vi "Dashboard Main.vi"() -> ()   [LabVIEW 2014]
uses:
  <vilib>/event_ctls.llb/eventvkey.ctl
  <vilib>/Rock Robotics/WPI/Dashboard/WPI_DashboardLogging Global.vi
  <vilib>/Utility/config.llb/Write Key (String).vi
  <vilib>/Utility/config.llb/Write Key (I32).vi
  <vilib>/Utility/config.llb/NI_LVConfig.lvlib
panel:
  in  "Toggle":bool
  in  "Enable":bool
  in  "Axis Cam IP":string
  out "Camera IP 3":string
  out "Camera IP 2":string
  out "Small":T1(plugin-control)
  in  "TCP":refnum<k5>
  in  "Rec Mode":enum32{"Stop", "Record", "Playback"}(radio)
  in  "Vision":u16(ring) items=["Camera Off", "USB Camera SW", "USB Camera HW", "IP Camera"]
  out "Camera IP":string
  out "Image Message":string="Timeout in Camera Communications"
  in  "Dashboard Tab":T2(tab)
  in  "Backwards Driving":bool
  out "fps 2":dbl format="%#.1g"
  out "Mbps 4":dbl format="%#.1g"
  out "Mbps 3":bool
  in  "Camera Settings":T3={"Frame Rate"=30, "Compression"=30, "Size"=1} {"Frame Rate" scale=1.0..30.0; "Size" items=["640x480", "320x240", "160x120"]}
  out "MotorChart R":cluster{"Numeric":dbl, "Numeric":dbl}(graph)
  out "MotorChart L":T4(graph)
  out "MotorSliders R":cluster{"MotorSlide1":dbl, "MotorSlide2":dbl} {"MotorSlide2" scale=-1.0..1.0 scale format="%#_2e"; "MotorSlide1" scale=-1.0..1.0 scale format="%#_2e"}
  out "MotorSliders L":T5 {"MotorSlide4 2" scale=0.0..14.0 scale format="%#_2e"; "MotorSlide2" scale=-1.0..1.0 scale format="%#_2e"; "MotorSlide1" scale=-1.0..1.0 scale format="%#_2e"}
  out "Gyro":dbl(knob) scale=0.0..360.0
  out "JS1 Z":dbl(slide) scale=-1.0..1.0 scale format="%#_2e"
  out "JS1 Graph":cluster{"X":dbl, "Y":dbl}[](graph)
  out "JS1 Buttons":T6
  out "JS2 Z":dbl(slide) scale=-1.0..1.0 scale format="%#_2e"
  out "JS2 Graph":cluster{"X":dbl, "Y":dbl}[](graph)
  out "JS2 Buttons":T6
  out "Mode":T7(ring)=enum."Auto Disabled"
  in  "DB Camera Config":bool
  out "fps":dbl format="%#.1g"
  out "Mbps":dbl format="%#.1g"
  out "Mbps 2":bool
  in  "DB/String 9":string
  in  "DB/String 8":string
  in  "DB/String 7":string
  in  "DB/String 6":string
  in  "DB/String 5":string
  in  "DB/String 4":string
  in  "DB/String 3":string
  in  "DB/String 2":string
  in  "DB/String 1":string
  in  "DB/String 0":string
  in  "DB/Slider 0":dbl(slide) scale=0.0..5.0
  in  "DB/Slider 1":dbl(slide) scale=0.0..5.0
  in  "DB/Slider 2":dbl(slide) scale=0.0..5.0
  in  "DB/Slider 3":dbl(slide) scale=0.0..5.0
  out "DB/LED 3":bool
  out "DB/LED 2":bool
  out "DB/LED 1":bool
  out "DB/LED 0":bool
  in  "DB/Button 3":bool
  in  "DB/Button 2":bool
  in  "DB/Button 1":bool
  in  "DB/Button 0":bool caption="New Name"
  in  "Test Slider":dbl(slide) scale=0.0..100.0 scale format="%#_3g"
  in  "On/Off":bool caption="Solenoid"
  in  "Test Name":u16(ring) items=["Select the test to run...", "Example Test", "-------------------------------", "List of tests is built in robot code.", "Replace with your own automated tests."]
  in  "Test Tree":string(tree)
  in  "Motor":cluster{"Value":dbl, "Enable":bool} {"Value" scale=-1.0..1.0 scale format="%#_3g"}
  out "Progress":T8 {"Test Progress" scale=0.0..100.0}
  in  "Rev/Fwd":cluster{"Forward":bool, "Reverse":bool}
  in  "Test Ring":u16(ring) items=["Monochrome", "Color"]
  in  "Listbox":i32(listbox)
  out "Tree":string(tree)
  out "Big":T1(plugin-control)
  out "Boolean":bool
  # "Left"
  # "Front"
  # "Right"
  # "Battery"
  # "This tab is a great place for autonomous settings and robot-specific values.\nPlace controls and indicators inside this tab and match name to\nDashboard Variables on robot. You can also delete this comment."
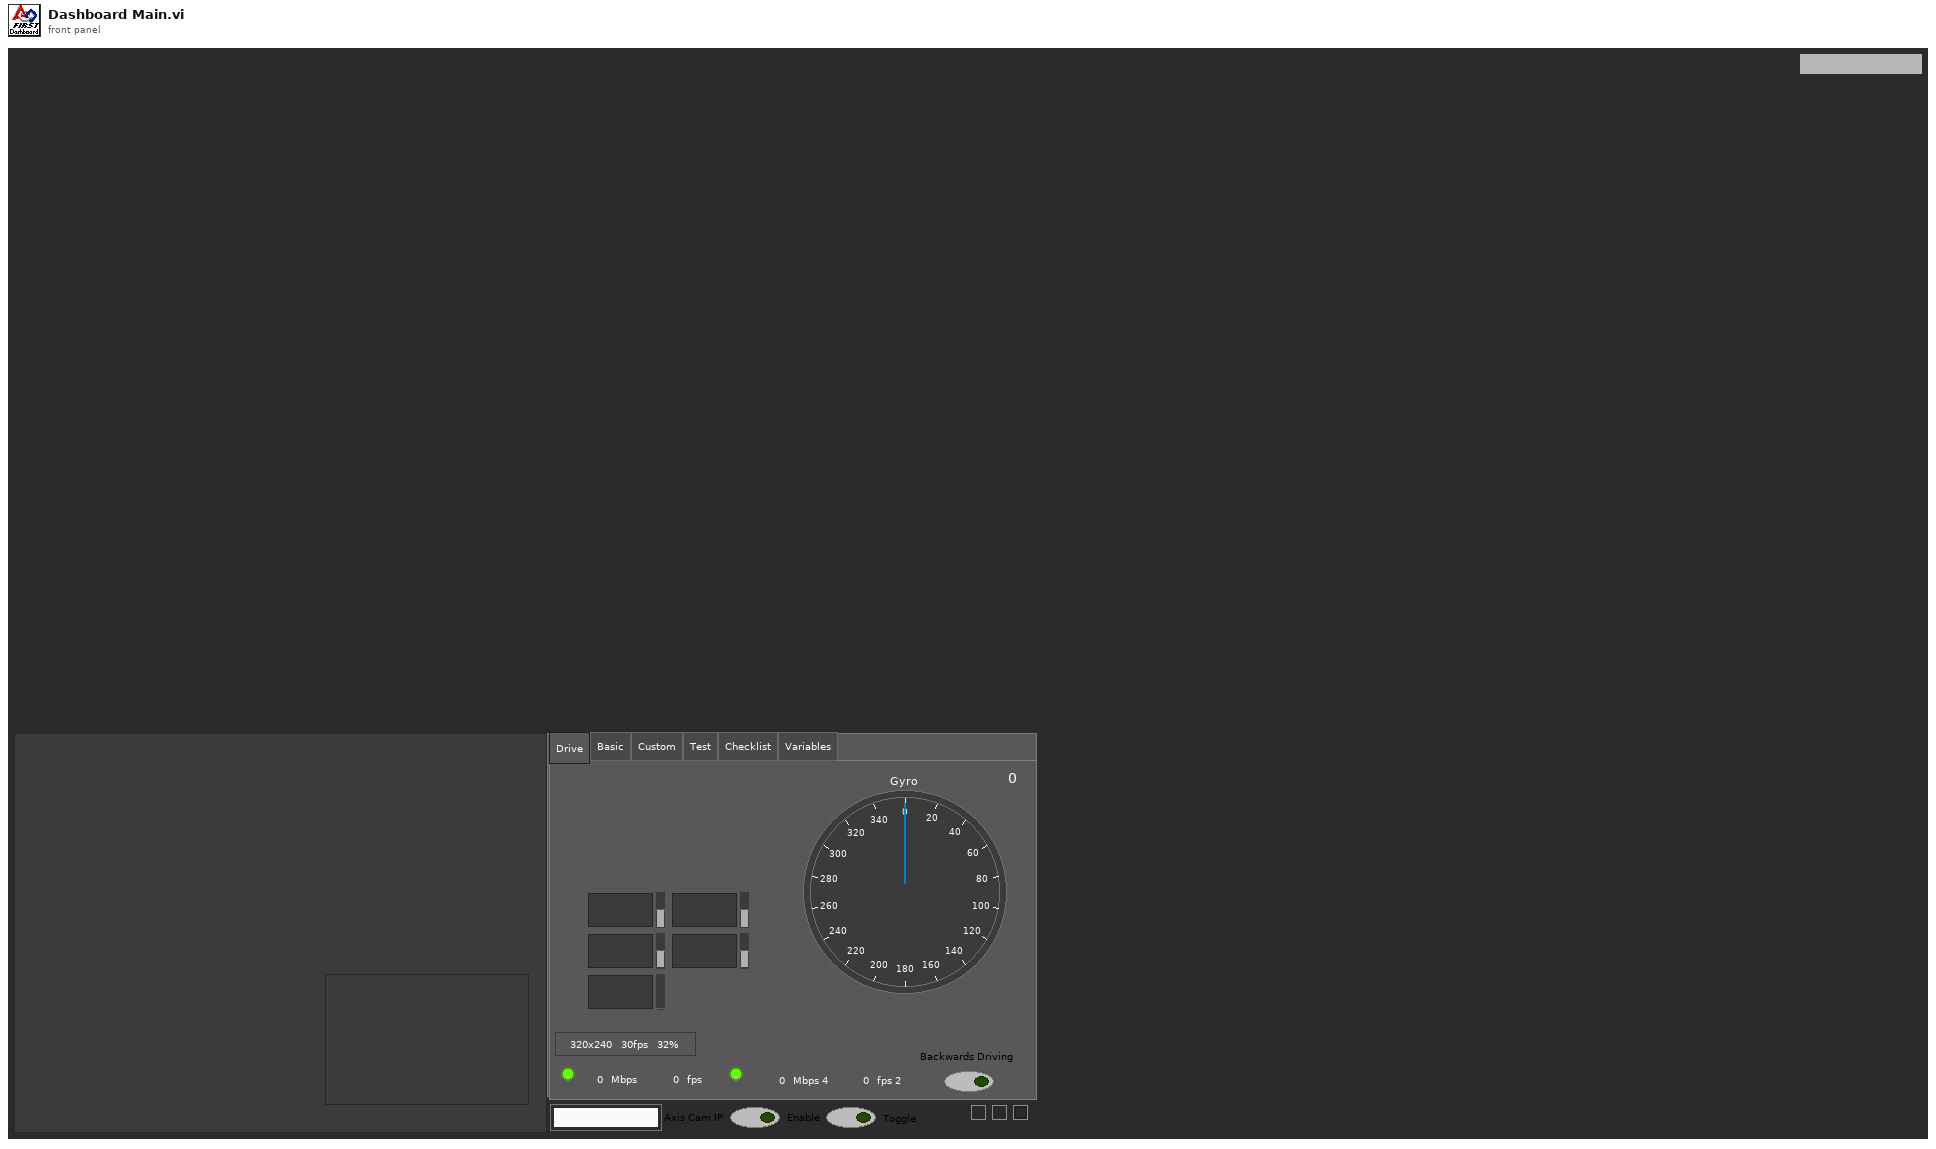
[diagram p1: front panel]
types:
  T1 = typedef "IMAQ Image.ctl" = refnum<image>
  T2 = enum32{"Drive", "Basic", "Custom", "Test", "Checklist", "Variables"}
  T3 = cluster{"Frame Rate":i32, "Compression":i32, "Size":u16}
  T4 = cluster{"Numeric":dbl, "Numeric":dbl, "Battery V":dbl}
  T5 = cluster{"MotorSlide1":dbl, "MotorSlide2":dbl, "MotorSlide4 2":dbl}
  T6 = cluster{bool, bool, bool, bool, bool, bool, bool, bool, bool, bool, bool, bool}
  T7 = enum8{"Tele-Op Disabled", "Tele-Op Enabled", "Auto Disabled", "Auto Enabled", "Test Disabled", "Test Enabled", "Disconnected", "No Code", "E-Stop"}
  T8 = cluster{"Test Progress":u8, "Test Progress Text":string}
  T9 = typedef "Image Type" = u32
  T10 = cluster{"Big":refnum<vi>, "Dashboard Tab":refnum<vi>, "Boolean":refnum<vi>, "Vision":refnum<vi>, "Rec Mode":refnum<vi>, "Test Slider":refnum<vi>, "On/Off ":refnum<vi>, "Test Ring":refnum<vi>, "Rev/Fwd":refnum<vi>, "Test Name":refnum<vi>, "Motor":refnum<vi>, "Progress":refnum<vi>, "CheckList":refnum<vi>, "Tree":refnum<vi>, "Test Tree":refnum<vi>}
  T11 = cluster{"Error Strings":string, "Disable Counts":cluster{u16, u16}, "Rail Faults":cluster{u16, u16, u16}, "Robot IP":string, "DB Mode":u8, "Event Info":cluster{"Name":string, "Type":u8, "Number":u16, "Replay":u8}, "Camera Addr":string}
  T12 = cluster{"Storage":cluster{"Disk Free":u64, "RAM Block":u32, "RAM free":u32}, "CPU Utilization":cluster{"CPU % ISR":sgl, "CPU % Time Crit":sgl, "CPU % Timed Str":sgl, "CPU % High":sgl, "CPU % Above":sgl, "CPU % Normal":sgl, "CPU % Low":sgl}, "CAN":cluster{"% Bus Utilization":sgl, "Bus Off Cnt":u32, "TX_FIFO Full Cnt":u32, "Receive Error Cnt":u8, "Transmit Error Cnt":u8}, "HID":cluster{"HID Outputs":u32, "Rumble Low":u16, "Rumble High":u16}[]}
  T13 = cluster{"Status bits":cluster{"Test Mode":bool, "Autonomous":bool, "Enabled":bool, "Code Start":bool, "Brownout":bool, "Reserved 2":bool, "Reserved 3":bool, "E-Stop":bool}, "Code Trace":cluster{"Disabled":bool, "TeleOp":bool, "Auto":bool, "Test":bool}, "Controller Type":enum16{"unknown", "cRIO", "roboRio"}, "Code?":enum16{"unknown", "noCode", "code"}, "Battery V":dbl}
  T14 = cluster{"Control Bits":cluster{"TestMode":bool, "Autonomous":bool, "Enabled":bool, "FMS Present":bool, bool, bool, bool, "E-Stop":bool}, "Team Station ":u8, "Countdown":sgl, "Joystick Values":cluster{"Axes":dbl[], "Buttons":bool[], "POVs":i16[]}[]}
  T15 = cluster{"Axes":dbl[], "Buttons":bool[], "POVs":i16[]}[]
  T16 = cluster{"Axes":dbl[], "Buttons":bool[], "POVs":i16[]}
  T17 = cluster{"Buttons[0]":bool, "Buttons[1]":bool, "Buttons[2]":bool, "Buttons[3]":bool, "Buttons[4]":bool, "Buttons[5]":bool, "Buttons[6]":bool, "Buttons[7]":bool, "Buttons[8]":bool, "Buttons[9]":bool, "Buttons[10]":bool, "Buttons[11]":bool}
  T18 = typedef "NI_LVConfig.lvlib/Config Data RefNum.ctl" = refnum<k1>
  T19 = cluster{"Operation":enum16{"Update", "Clear"}, "Color Box":u32}[]
  T20 = typedef "eventvkey.ctl" = enum16{"ASCII", "Enter", "Return", "Shift", "Ctrl", "Alt", "Cmd", "Opt", "Caps", "NumLock", "Clear", "Break", "Up", "Down", "Left", "Right", "Insert", "Delete", "Home", "End", "PageUp", "PageDown", "Escape", "Help", "Pause", "ScrollLock", "F1", "F2", "F3", "F4", "F5", "F6", "F7", "F8", "F9", "F10", "F11", "F12", "F13", "F14", "F15", "F16", "F17", "F18", "F19", "F20", "F21", "F22", "F23", "F24", "Play", "VolumeUp", "VolumeDown", "Mute", "Two Byte Char"}
  T21 = cluster{"Image Size":bool, "Image Type":bool, "Pixel Value":bool, "ROI Information":bool, "Zoom Factor":bool}
  T22 = enum8{"Enabled", "Disabled", "Disabled and Grayed Out"}
  T23 = cluster{"Operation":enum16{"Update", "Clear"}, "Color Box":u32}
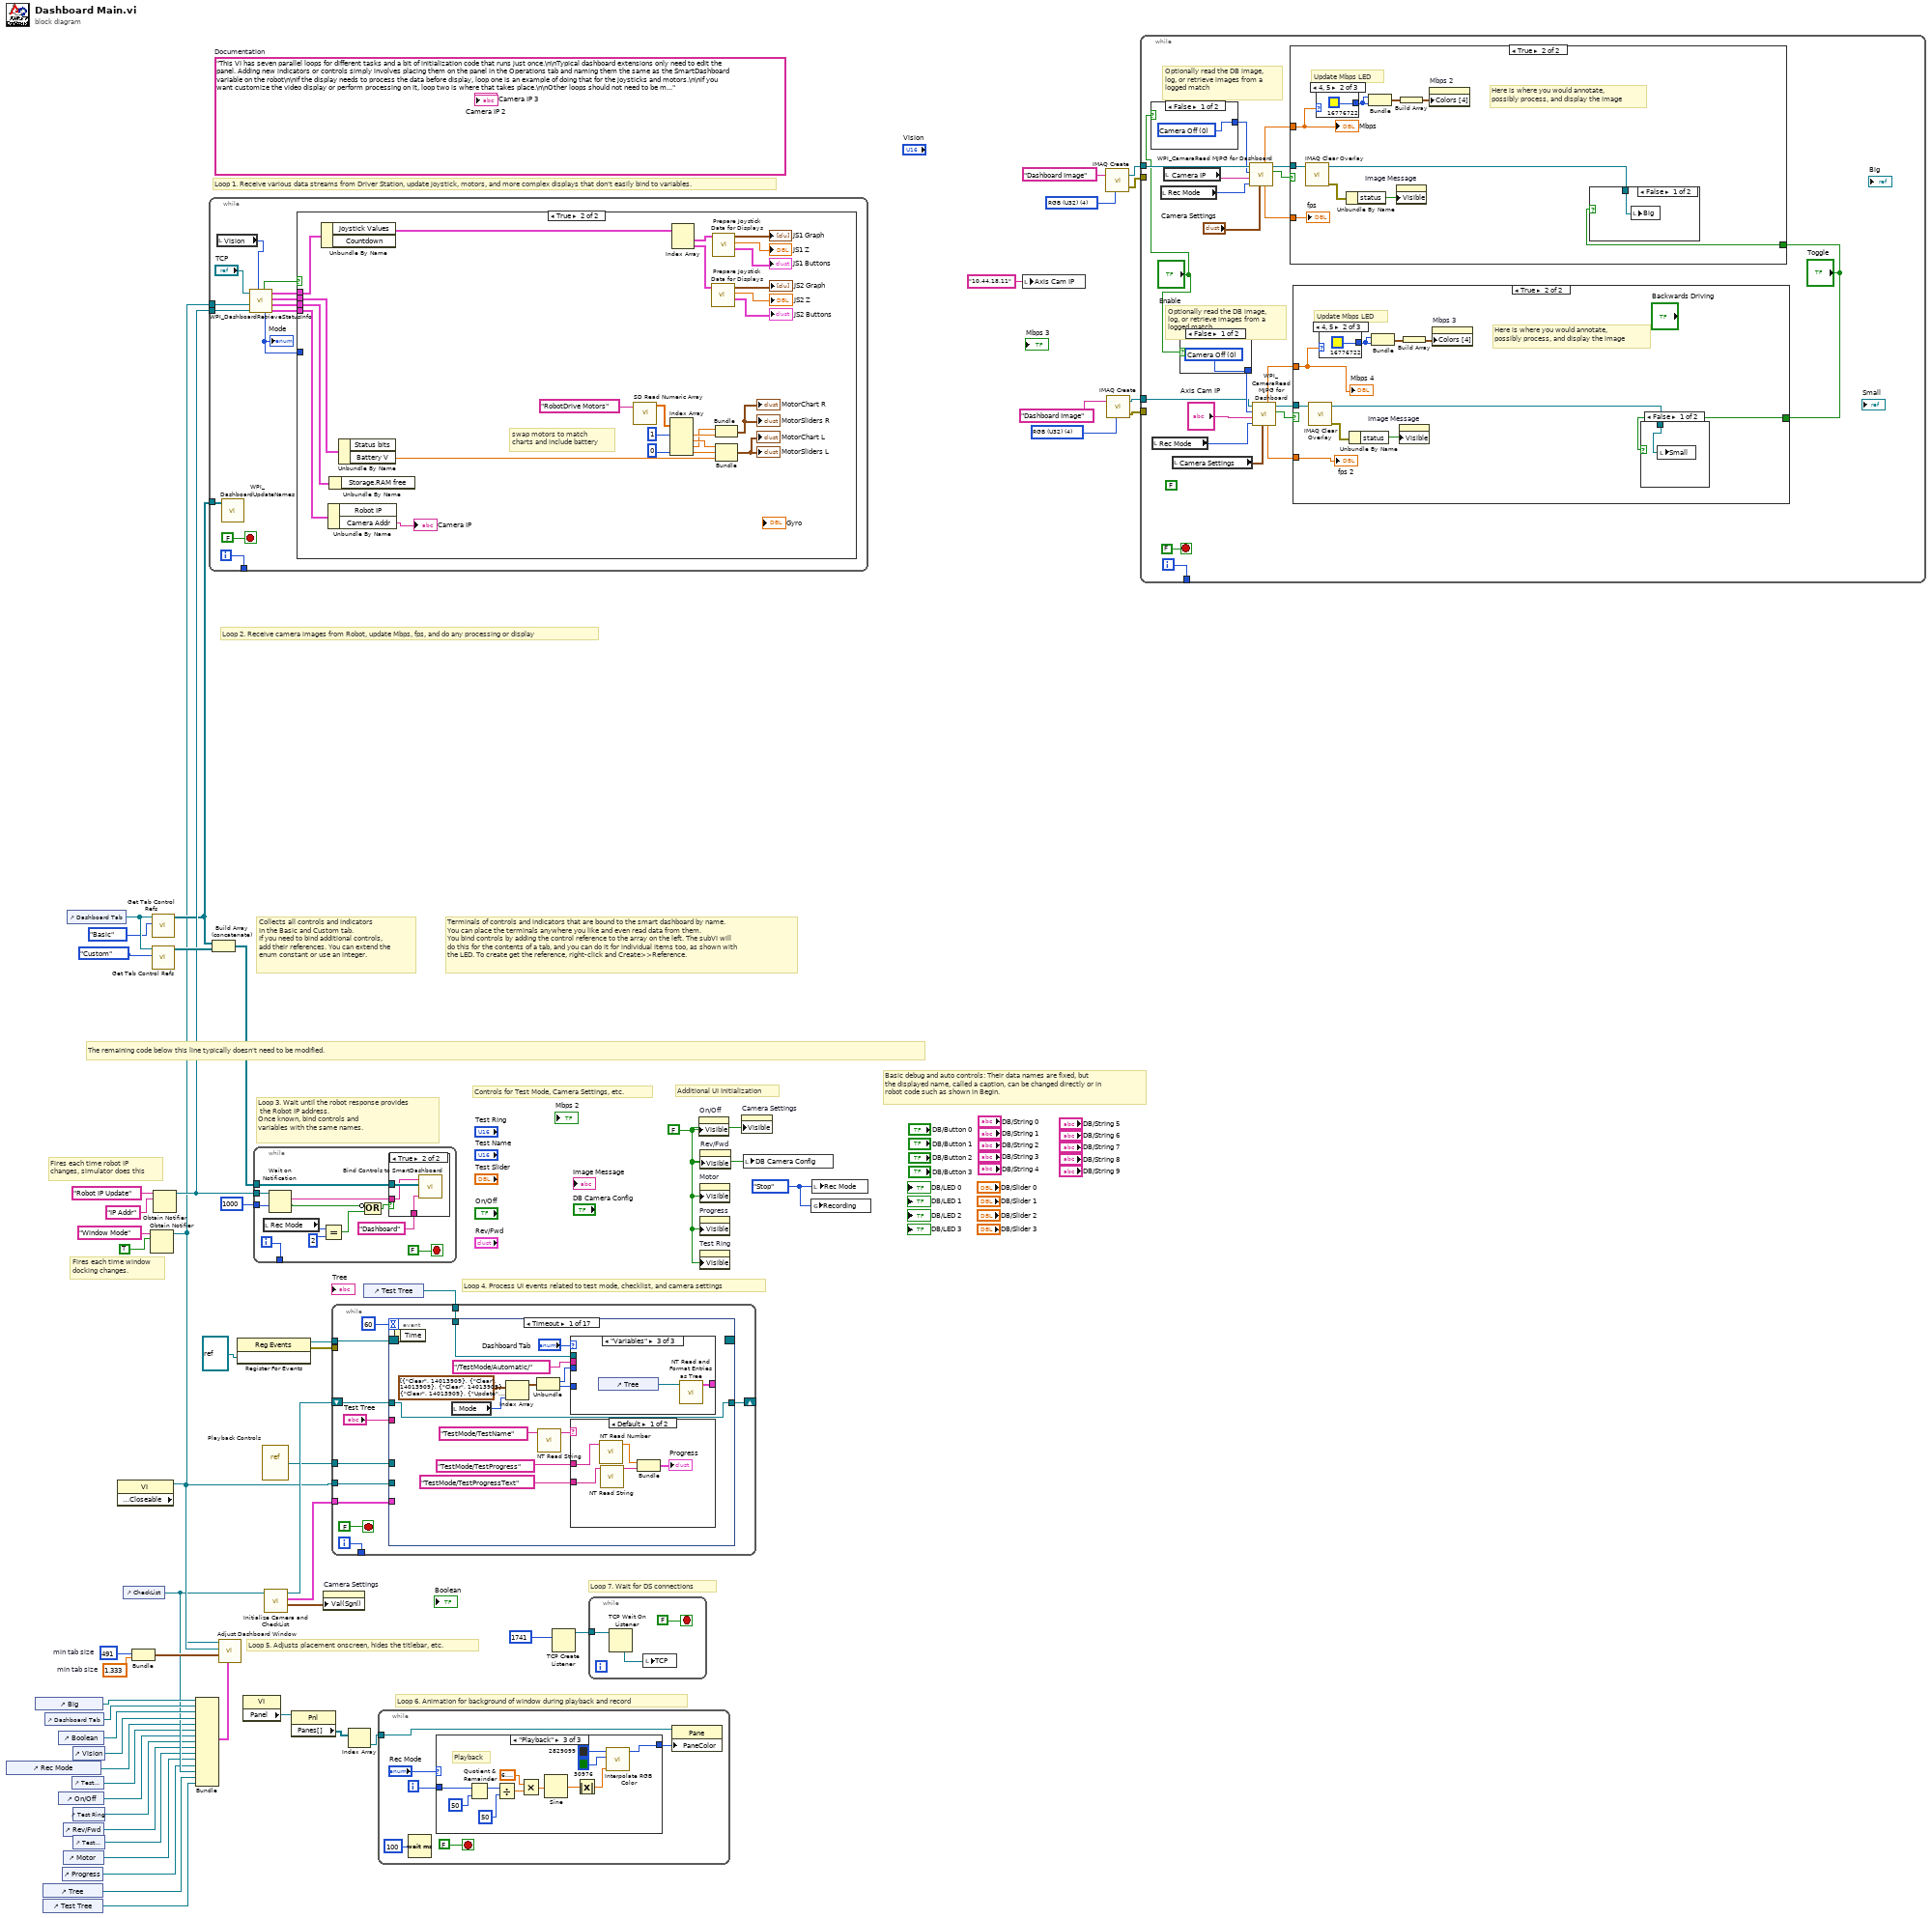
[diagram p0: block diagram]
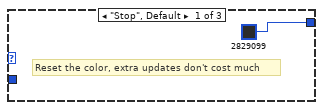
[diagram p3: hidden frame]
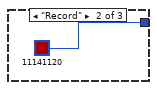
[diagram p4: hidden frame]
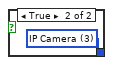
[diagram p6: hidden frame]
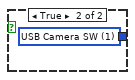
[diagram p7: hidden frame]
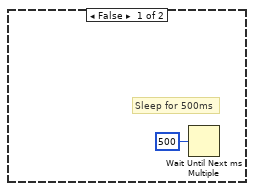
[diagram p8: hidden frame]
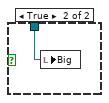
[diagram p9: hidden frame]
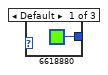
[diagram p10: hidden frame]
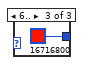
[diagram p11: hidden frame]
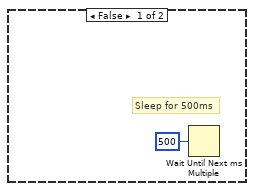
[diagram p12: hidden frame]
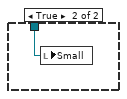
[diagram p13: hidden frame]
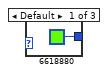
[diagram p14: hidden frame]
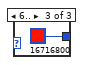
[diagram p15: hidden frame]
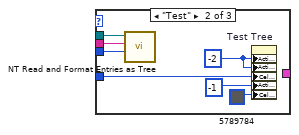
[diagram p17: hidden frame]
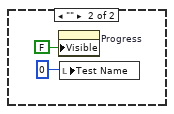
[diagram p18: hidden frame]
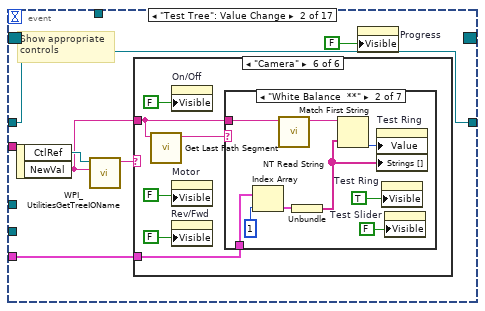
[diagram p19: hidden frame]
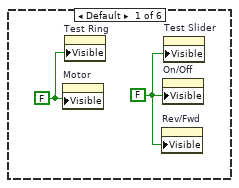
[diagram p20: hidden frame]
diagram:
  w4 = T9 4 items=["Grayscale (U8)", "Grayscale (I16)", "Grayscale (SGL)", "Complex (CSG)", "RGB (U32)", "HSL (U32)", "RGB (U64)"] ("Image Type")
  w29 = 491  # min tab size
  w28 = 1.333  # min tab size
  w37 = enum32{"Stop", "Record", "Playback"}."Stop" ("Rec Mode")
  w11 = FALSE ("Visible")
  (unwired) "This VI has seven parallel loops for different tasks and a bit of initialization code that runs just once.\n\nTypical dashboard extensions only need to edit the panel. Adding new indicators or controls simply involves placing them on the panel in the Operations tab and naming them the same as the SmartDashboard variable on the robot\n\nIf the display needs to process the data before display, loop one is an example of doing that for the joysticks and motors.\n\nIf you want customize the video display or perform processing on it, loop two is where that takes place.\n\nOther loops should not need to be modified. They are pretty standard, and document the task they perform."  # Documentation
  w57 = T9 4 items=["Grayscale (U8)", "Grayscale (I16)", "Grayscale (SGL)", "Complex (CSG)", "RGB (U32)", "HSL (U32)", "RGB (U64)"] ("Image Type")
  # "Loop 7. Wait for DS connections"
  # "Basic debug and auto controls: Their data names are fixed, but\nthe displayed name, called a caption, can be changed directly or in\nrobot code such as shown in Begin."
  # "Controls for Test Mode, Camera Settings, etc."
  # "Additional UI Initialization"
  # "Loop 6. Animation for background of window during playback and record"
  # "Fires each time robot IP\nchanges, simulator does this"
  # "Fires each time window\ndocking changes."
  # "Collects all controls and indicators\nin the Basic and Custom tab.\nIf you need to bind additional controls,\nadd their references. You can extend the\nenum constant or use an integer."
  # "The remaining code below this line typically doesn't need to be modified."
  # "Loop 4. Process UI events related to test mode, checklist, and camera settings"
  # "Terminals of controls and indicators that are bound to the smart dashboard by name.\nYou can place the terminals anywhere you like and even read data from them.\nYou bind controls by adding the control reference to the array on the left. The subVI will\ndo this for the contents of a tab, and you can do it for individual items too, as shown with\nthe LED. To create get the reference, right-click and Create>>Reference."
  # "Loop 3. Wait until the robot response provides\n the Robot IP address.\nOnce known, bind controls and\nvariables with the same names."
  # "Loop 5. Adjusts placement onscreen, hides the titlebar, etc."
  # "Loop 1. Receive various data streams from Driver Station, update joystick, motors, and more complex displays that don't easily bind to variables."
  # "Loop 2. Receive camera images from Robot, update Mbps, fps, and do any processing or display"
  n1 = control-ref of="Rec Mode"() -> (w17:refnum<vi>)
  n2 = control-ref of="Big"() -> (w32:refnum<vi>)
  n3 = control-ref of="Tree"() -> (w21:refnum<vi>)
  n4 = control-ref of="Test Tree"() -> (w20:refnum<vi>)
  n5 = control-ref of="Dashboard Tab"() -> (w31:refnum<vi>)
  n6 = control-ref of="Boolean"() -> (w26:refnum<vi>)
  n7 = control-ref of="On/Off"() -> (w15:refnum<vi>)
  n8 = control-ref of="Progress"() -> (w12:refnum<vi>)
  n9 = control-ref of="Rev/Fwd"() -> (w13:refnum<vi>)
  n10 = control-ref of="Motor"() -> (w18:refnum<vi>)
  n11 = control-ref of="Dashboard Tab"() -> (w35:refnum<vi>)
  n12 = control-ref of="Test Slider"() -> (w16:refnum<vi>)
  n13 = control-ref of="Vision"() -> (w30:refnum<vi>)
  n14 = control-ref of="Test Ring"() -> (w14:refnum<vi>)
  n15 = control-ref of="Test Name"() -> (w19:refnum<vi>)
  n16 = property class="VI" props=["Front Panel.Closeable"]() -> (reference out=w36:refnum<vi>)  [unwired: 2 in, 2 out]
  n17 = control-ref of="CheckList"() -> (w22:refnum<vi>)
  n18 = Bundle("min tab size"=w29, "min tab size"=w28) -> (w27:cluster{"min tab size":i32, "min tab size":dbl})  [unwired: 1 in]
  n19 = Obtain Notifier(name (unnamed)="Window Mode", notification data type=TRUE) -> (notifier out=w8:refnum<notifier>)  [unwired: 2 in, 2 out]
  n20 = call <vilib>:"Get Tab Control Refs.vi"("Page Index"=T2."Basic" ("Dashboard Tab"), "TabControl in"=w35) -> ("ControlsOnPage"=w9:refnum<vi>[])  [unwired: 9 in]
  n21 = call <vilib>:"Get Tab Control Refs.vi"("Page Index"=T2."Custom" ("Dashboard Tab"), "TabControl in"=w35) -> ("ControlsOnPage"=w34:refnum<vi>[])  [unwired: 9 in]
  n22 = Obtain Notifier(name (unnamed)="Robot IP Update", notification data type="IP Addr" ("name (unnamed)")) -> (notifier out=w10:refnum<notifier>)  [unwired: 2 in, 2 out]
  n23 = Bundle("Big"=w32, "Dashboard Tab"=w31, "Boolean"=w26, "Vision"=w30, "Rec Mode"=w17, "Test Slider"=w16, "On/Off"=w15, "Test Ring"=w14, "Rev/Fwd"=w13, "Test Name"=w19, "Motor"=w18, "Progress"=w12, "CheckList"=w22, "Tree"=w21, "Test Tree"=w20) -> (w23:T10)  [unwired: 1 in]
  n24 = while {
    tunnel: [w69] -> _
    tunnel: w10 -> [w63]
    tunnel: w9 -> [w62]
    tunnel: w8 -> [w58]
    i -> [w69]
    stop <- FALSE stop-if-true
    n25 = local read "Vision"() -> (w60:u16)
    n26 = call <vilib>:"WPI_DashboardUpdateNames.vi"("Controls on Tab"=w62) -> ()  [unwired: 11 in]
    n27 = call <vilib>:"WPI_DashboardRetrieveStatusInfo.vi"("Vision"=w60, "Binding Refnum"=w63, "Window Mode Notifier"=w58, "TCP Cnx"="TCP") -> ("Power and Errors"=w64:T11, "Robot Metrics"=w67:T12, "Status Info"=w68:T13, "Control Info"=w65:T14, "Robot Mode"=w61:T7, "Process?"=w66:bool)  [unwired: 2 in]
    "Mode" <- w61
    n28 = case shown="True" w66 {
      tunnel: w68 -> [_ w95]
      tunnel: w67 -> [_ w94]
      tunnel: w65 -> [_ w93]
      tunnel: w64 -> [_ w92]
      tunnel: w61 -> [_ _]
      frame False {
      }
      frame True {
        # "swap motors to match\ncharts and include battery"
        n29 = Unbundle By Name(w93) -> ("Joystick Values"=w80:T15)  [unwired: 1 out]
        n30 = Unbundle By Name(w92) -> ("Camera Addr"=→"Camera IP":string)  [unwired: 1 out]
        n31 = Unbundle By Name(w94) -> ()  [unwired: 1 out]
        n32 = Unbundle By Name(w95) -> ("Battery V"=w81:dbl)  [unwired: 1 out]
        n33 = call <vilib>:"SD Read Numeric Array.vi"("Name"="RobotDrive Motors") -> ("Numeric Array"=w83:dbl[])  [unwired: 8 in, 2 out]
        n34 = Index Array(array=w83, index #1=1, index #4=0) -> (element #1=w87:dbl, element #2=w88:dbl, element #3=w86:dbl, element #4=w91:dbl)  [unwired: 2 in]
        n35 = Index Array(array=w80) -> (element #1=w79:T16, element #2=w74:T16)  [unwired: 2 in]
        n36 = call "Prepare Joystick Data for Displays.vi"("Joystick Values"=w74) -> ("Buttons"=→"JS2 Buttons":T17, "Z Axis"=→"JS2 Z":dbl, "Cartesian Data"=→"JS2 Graph":cluster{"X axis":dbl, "X axis":dbl}[])  [unwired: 8 in]
        n37 = call "Prepare Joystick Data for Displays.vi"("Joystick Values"=w79) -> ("Buttons"=→"JS1 Buttons":T17, "Z Axis"=→"JS1 Z":dbl, "Cartesian Data"=→"JS1 Graph":cluster{"X axis":dbl, "X axis":dbl}[])  [unwired: 8 in]
        n38 = Bundle("Numeric"=w86, "Numeric"=w87) -> (→"MotorChart R" →"MotorSliders R":cluster{"Numeric":dbl, "Numeric":dbl})  [unwired: 1 in]
        n39 = Bundle("Numeric"=w88, "Numeric"=w91, "Battery V"=w81) -> (→"MotorChart L" →"MotorSliders L":T4)  [unwired: 1 in]
      }
    }
  }
  n40 = Build Array (concatenate)(w9, w34) -> (w33:refnum<vi>[])
  n41 = call "Adjust Dashboard Window.vi"("Sizing Refnums"=w23, "Size Constraints"=w27, "VI"=w36, "Notifier in"=w8) -> ()  [unwired: 8 in]
  n42 = register-events(refnum<vi> refnum) -> (reference out=w41:refnum<event-registration>, error out=w40:errorcluster)  [unwired: 2 in]
  n43 = property class="VI"() -> ("Panel"=w44:refnum<vi>)  [unwired: 2 in, 2 out]
  n44 = while {
    tunnel: w33 -> [w107]
    tunnel: w10 -> [w105]
    tunnel: [w103] -> _
    tunnel: u32 1000 ("milliseconds to wait") -> [w102]
    i -> [w103]
    stop <- FALSE stop-if-true
    n45 = local read "Rec Mode"() -> (w98:enum32{"Stop", "Record", "Playback"})
    n46 = Wait on Notification(notifier=w105, timeout in ms (-1)=w102) -> (notification=w104:string, timed out?=w100:bool)  [unwired: 2 in, 2 out]
    n47 = Equal?(x=w98, y=u16 2 ("Rec Mode")) -> (x = y?=w99:bool)
    n48 = Compound Arithmetic op=OR(invert w100, w99) -> (w101:bool)
    n49 = case shown="True" w101 {
      tunnel: w107 -> [_ w110]
      tunnel: w104 -> [_ w109]
      tunnel: "Dashboard" -> [_ w108]
      frame False {
      }
      frame True {
        n50 = call <vilib>:"Bind Controls to SmartDashboard.vi"("Client Name"=w108, "Bound Control Refs"=w110, "Server IP Address"=w109) -> ()  [unwired: 9 in]
      }
    }
  }
  n51 = vi-ref "Playback Controls.vi"() -> (w42:refnum<vi>)
  n52 = call "Initialize Camera and CheckList.vi"("ListBox in"=w22) -> ("Cluster"=w48:cluster{"value":i32, "value":i32, "index":i32}, "Array"=w49:cluster{string[]}[], "File Refnum"=w47:T18)  [unwired: 8 in]
  n53 = property class="Pnl"(reference=w44) -> ("Panes[]"=w45:refnum<vi>[])  [unwired: 1 in, 2 out]
  n54 = property on="Camera Settings" class="Clust (strict)"("Val(Sgnl)"=w48) -> ()  [unwired: 2 in, 2 out]
  n55 = Index Array(array=w45) -> (element=w43:refnum<vi>)  [unwired: 1 in]
  n56 = control-ref of="Test Tree"() -> (w46:refnum<vi>)
  n57 = while {
    tunnel: w49 -> [w118]
    shift-right: [w117] -> _
    shift-left: w47 -> [w116]
    tunnel: [w115] -> _
    tunnel: w46 -> [w114]
    tunnel: w42 -> [w113]
    tunnel: w41 -> [w112]
    tunnel: w40 -> [_]
    tunnel: w36 -> [w111]
    i -> [w115]
    stop <- FALSE stop-if-true
    n58 = event shown="[0] Timeout" {
      selector: w112 -> [_ _ _ _ _ _ _ _ _ _ _ _ _ _ _ _ _]
      dyn-events: [_ _ _ _ _ _ _ _ _ _ _ _ _ w356 _ _ _] -> _
      timeout: u32 60 ("milliseconds to wait") -> [_ _ _ _ _ _ _ _ _ _ _ _ _ _ _ _ _]
      tunnel: w114 -> [w130 _ _ _ _ _ _ _ _ _ _ _ _ _ _ _ _]
      tunnel: "Test Tree" -> [_ _ _ _ _ _ _ _ w325 w333 w335 w339 w347 _ _ _ _]
      tunnel: w118 -> [_ w152 _ _ _ _ w289 w319 _ _ _ _ _ _ _ _ _]
      tunnel: [w126 w151 w250 w255 w263 w275 w288 w312 w324 w331 w334 w338 w346 w358 w372 w373 w383] -> w117
      tunnel: w116 -> [w126 w151 w250 w255 w263 w275 w287 w312 w324 w331 w334 w338 w346 w358 w372 w373 w383]
      tunnel: w113 -> [_ _ _ _ _ _ _ _ _ _ _ _ _ w359 _ w376 _]
      tunnel: w111 -> [_ _ _ _ _ _ _ _ _ _ _ _ _ w354 _ _ _]
      event Timeout {
        n59 = event-data() -> ()  [unwired: 1 in, 1 out]
        n60 = local read "Mode"() -> (w129:T7)
        n61 = Index Array(array=T19 [{"Operation"=enum."Clear", "Color Box"=14013909}, {"Operation"=enum."Clear", "Color Box"=14013909}, {"Operation"=enum."Clear", "Color Box"=14013909}, {"Operation"=enum."Clear", "Color Box"=14013909}, {"Operation"=enum."Update", "Color Box"=14013909}, {"Operation"=enum."Update", "Color Box"=16777215}, {"Operation"=enum."Clear", "Color Box"=14013909}, {"Operation"=enum."Clear", "Color Box"=14013909}, {"Operation"=enum."Clear", "Color Box"=14013909}], index=w129) -> (element=w124:T23)
        n62 = Unbundle(w124) -> ("Operation"=w123:enum16{"Update", "Clear"}, "Color Box"=w122:u32)
        n63 = call <vilib>:"NT Read String.vi"("Name"="TestMode/TestName") -> ("String"=w133:string)  [unwired: 9 in, 1 out]
        n64 = case shown="\"Variables\"" "Dashboard Tab" {
          tunnel: w130 -> [_ w141 _]
          tunnel: "/TestMode/Automatic/" ("Name Pattern") -> [_ w140 _]
          tunnel: w123 -> [_ w139 _]
          tunnel: [_ _ w143] -> _
          tunnel: w122 -> [_ w135 _]
          frame "Custom", Default {
          }
          frame "Test" {
            w138 = -2 ("Active Item:Row Number")
            n65 = call <vilib>:"NT Read and Format Entries as Tree.vi"("Operation"=w139, "Name Pattern"=w140, "Tree Refnum"=w141) -> ()  [unwired: 7 in, 2 out]
            n66 = property on="Test Tree" class="Tree (strict)"("Active Item Row Number"=w138, "ActiveColNum"=w138, "CellBG"=w135, "Active Item Row Number"=-1 ("Active Item:Row Number"), "CellBG"=u32 5789784 ("Color Box")) -> ()  [unwired: 2 in, 2 out]
          }
          frame "Variables" {
            n67 = control-ref of="Tree"() -> (w142:refnum<vi>)
            n68 = call <vilib>:"NT Read and Format Entries as Tree.vi"("Tree Refnum"=w142) -> ("Formatted Strings"=w143:cluster{"Name":string, "Value":string}[])  [unwired: 9 in, 1 out]
          }
        }
        n69 = case shown="Default" w133 {
          tunnel: "TestMode/TestProgress" ("Name") -> [w145 _]
          tunnel: "TestMode/TestProgressText" ("Name") -> [w144 _]
          frame Default {
            n70 = call <vilib>:"NT Read Number.vi"("Name"=w145) -> ("Numeric"=w146:dbl)  [unwired: 9 in, 1 out]
            n71 = call <vilib>:"NT Read String.vi"("Name"=w144) -> ("String"=w147:string)  [unwired: 9 in, 1 out]
            n72 = Bundle("Numeric"=w146, "String"=w147) -> (→"Progress":cluster{"Numeric":dbl, "String":string})  [unwired: 1 in]
          }
          frame "" {
            n73 = property on="Progress" class="Clust (strict)"("Visible"=FALSE) -> ()  [unwired: 2 in, 2 out]
            n74 = local write "Test Name"(u16 0) -> ()
          }
        }
      }
      event "Test Tree": Value Change {
        # "Show appropriate\ncontrols"
        n75 = event-data() -> ("CtlRef"=w155:refnum<vi>, "NewVal"=w153:string)  [unwired: 1 in]
        n76 = call <vilib>:"WPI_UtilitiesGetTreeIOName.vi"("NewVal"=w153, "TreeControl in"=w155) -> ("I/O Name"=w156:string)  [unwired: 9 in]
        n77 = case shown="\"Camera\"" w156 {
          selector: w156 -> [_ w163 _ w181 w190 _]
          tunnel: w153 -> [_ _ w178 w180 _ w197]
          tunnel: w152 -> [_ _ _ _ _ w196]
          frame Default {
            w158 = FALSE ("Visible")
            w157 = FALSE ("Visible")
            n78 = property on="Motor" class="Clust (strict)"("Visible"=w157) -> ()  [unwired: 2 in, 2 out]
            n79 = property on="Test Ring" class="Ring (strict)"("Visible"=w157) -> ()  [unwired: 2 in, 2 out]
            n80 = property on="Rev/Fwd" class="Clust (strict)"("Visible"=w158) -> ()  [unwired: 2 in, 2 out]
            n81 = property on="On/Off" class="Bool (strict)"("Visible"=w158) -> ()  [unwired: 2 in, 2 out]
            n82 = property on="Test Slider" class="Slide (strict)"("Visible"=w158) -> ()  [unwired: 2 in, 2 out]
          }
          frame "Motor", "PWM" {
            w164 = FALSE ("Visible")
            n83 = case shown="\"Motor\", Default" w163 {
              tunnel: [1.0 ("Value") -1.0 ("Value")] -> w162
              tunnel: [255.0 ("Value") 1.0 ("Value")] -> w161
              tunnel: [128.0 ("Value") 0.0 ("Value")] -> w160
              tunnel: [64.0 ("Value") 0.5 ("Value")] -> w159
              frame "PWM" {
              }
              frame "Motor", Default {
              }
            }
            n84 = property on="Motor" class="Clust (strict)"("Visible"=TRUE) -> ()  [unwired: 2 in, 2 out]
            n85 = property on="Value" class="Slide (strict)"("Value"=w160, "Scale.Minimum"=w162, "Scale.Maximum"=w161, "Scale.Increment"=w159) -> ()  [unwired: 2 in, 2 out]
            n86 = property on="On/Off" class="Bool (strict)"("Visible"=w164) -> ()  [unwired: 2 in, 2 out]
            n87 = property on="Test Slider" class="Slide (strict)"("Visible"=w164) -> ()  [unwired: 2 in, 2 out]
            n88 = property on="Test Ring" class="Ring (strict)"("Visible"=w164) -> ()  [unwired: 2 in, 2 out]
            n89 = property on="Rev/Fwd" class="Clust (strict)"("Visible"=w164) -> ()  [unwired: 2 in, 2 out]
          }
          frame "Servo" {
            w176 = FALSE ("Visible")
            n90 = call <vilib>:"NT Read Number.vi"("Name"=w178) -> ("Numeric"=w177:dbl)  [unwired: 9 in, 1 out]
            n91 = property on="Test Slider" class="Slide (strict)"("Visible"=TRUE, "Scale.Maximum"=170.0 ("Scale.Range:Maximum")) -> ()  [unwired: 2 in, 2 out]
            n92 = local write "Test Slider"(w177) -> ()
            n93 = property on="Motor" class="Clust (strict)"("Visible"=w176) -> ()  [unwired: 2 in, 2 out]
            n94 = property on="Rev/Fwd" class="Clust (strict)"("Visible"=w176) -> ()  [unwired: 2 in, 2 out]
            n95 = property on="On/Off" class="Bool (strict)"("Visible"=w176) -> ()  [unwired: 2 in, 2 out]
            n96 = property on="Test Ring" class="Ring (strict)"("Visible"=w176) -> ()  [unwired: 2 in, 2 out]
          }
          frame "Relay", "Solenoid" {
            w179 = FALSE ("Visible")
            n97 = property on="Motor" class="Clust (strict)"("Visible"=w179) -> ()  [unwired: 2 in, 2 out]
            n98 = property on="Test Slider" class="Slide (strict)"("Visible"=w179) -> ()  [unwired: 2 in, 2 out]
            n99 = Search and Replace String(input string=w180, search string="/Value  **", replace string="/Direction") -> (result string=w186:string)  [unwired: 5 in, 3 out]
            n100 = property on="Test Ring" class="Ring (strict)"("Visible"=w179) -> ()  [unwired: 2 in, 2 out]
            n101 = call <vilib>:"NT Read String.vi"("Name"=w186) -> ("String"=w184:string)  [unwired: 9 in, 1 out]
            n102 = Equal?(x="Both directions", y=w184) -> (x = y?=w182:bool)
            n103 = Not(x=w182) -> (.not. x?=w183:bool)
            n104 = property on="Rev/Fwd" class="Clust (strict)"("Visible"=w182) -> ()  [unwired: 2 in, 2 out]
            n105 = property on="On/Off" class="Bool (strict)"("Visible"=w183, "Caption.Text"=w181) -> ()  [unwired: 2 in, 2 out]
          }
          frame "Compressor", "Digital Out" {
            w189 = FALSE ("Visible")
            # "Get direction and finish"
            n106 = property on="Motor" class="Clust (strict)"("Visible"=w189) -> ()  [unwired: 2 in, 2 out]
            n107 = property on="Test Slider" class="Slide (strict)"("Visible"=w189) -> ()  [unwired: 2 in, 2 out]
            n108 = property on="Test Ring" class="Ring (strict)"("Visible"=w189) -> ()  [unwired: 2 in, 2 out]
            n109 = property on="On/Off" class="Bool (strict)"("Visible"=TRUE, "Caption.Text"=w190) -> ()  [unwired: 2 in, 2 out]
            n110 = property on="Rev/Fwd" class="Clust (strict)"("Visible"=FALSE) -> ()  [unwired: 2 in, 2 out]
          }
          frame "Camera" {
            n111 = call <vilib>:"Get Last Path Segment.vi"("String in"=w197) -> ("String out"=w198:string)  [unwired: 10 in]
            n112 = property on="On/Off" class="Bool (strict)"("Visible"=FALSE) -> ()  [unwired: 2 in, 2 out]
            n113 = property on="Motor" class="Clust (strict)"("Visible"=FALSE) -> ()  [unwired: 2 in, 2 out]
            n114 = property on="Rev/Fwd" class="Clust (strict)"("Visible"=FALSE) -> ()  [unwired: 2 in, 2 out]
            n115 = case shown="\"White Balance  **\"" w198 {
              tunnel: w197 -> [w204 w213 w222 w231 w240 _ w246]
              tunnel: w196 -> [w202 w210 w219 w228 w237 _ _]
              frame "Size  **" {
                n116 = Index Array(array=w202) -> (element=w201:cluster{string[]})  [unwired: 1 in]
                n117 = call <vilib>:"NT Read String.vi"("Name"=w204) -> ("String"=w203:string)  [unwired: 9 in, 1 out]
                n118 = Unbundle(w201) -> (w199:string[])
                n119 = Match First String(2:w199, 3:w203) -> (0:w200:i32)  [unwired: 1 out]
                n120 = property on="Test Ring" class="Ring (strict)"("Value"=w200, "Strings []"=w199) -> ()  [unwired: 2 in, 2 out]
                n121 = property on="Test Ring" class="Ring (strict)"("Visible"=TRUE) -> ()  [unwired: 2 in, 2 out]
                n122 = property on="Test Slider" class="Slide (strict)"("Visible"=FALSE) -> ()  [unwired: 2 in, 2 out]
              }
              frame "White Balance  **" {
                n123 = Index Array(array=w210, index=1) -> (element=w211:cluster{string[]})
                n124 = call <vilib>:"NT Read String.vi"("Name"=w213) -> ("String"=w212:string)  [unwired: 9 in, 1 out]
                n125 = Unbundle(w211) -> (w208:string[])
                n126 = Match First String(2:w208, 3:w212) -> (0:w207:i32)  [unwired: 1 out]
                n127 = property on="Test Ring" class="Ring (strict)"("Value"=w207, "Strings []"=w208) -> ()  [unwired: 2 in, 2 out]
                n128 = property on="Test Ring" class="Ring (strict)"("Visible"=TRUE) -> ()  [unwired: 2 in, 2 out]
                n129 = property on="Test Slider" class="Slide (strict)"("Visible"=FALSE) -> ()  [unwired: 2 in, 2 out]
              }
              frame "Exposure  **" {
                n130 = Index Array(array=w219, index=2) -> (element=w220:cluster{string[]})
                n131 = call <vilib>:"NT Read String.vi"("Name"=w222) -> ("String"=w221:string)  [unwired: 9 in, 1 out]
                n132 = Unbundle(w220) -> (w216:string[])
                n133 = Match First String(2:w216, 3:w221) -> (0:w217:i32)  [unwired: 1 out]
                n134 = property on="Test Ring" class="Ring (strict)"("Value"=w217, "Strings []"=w216) -> ()  [unwired: 2 in, 2 out]
                n135 = property on="Test Ring" class="Ring (strict)"("Visible"=TRUE) -> ()  [unwired: 2 in, 2 out]
                n136 = property on="Test Slider" class="Slide (strict)"("Visible"=FALSE) -> ()  [unwired: 2 in, 2 out]
              }
              frame "Exposure Priority  **" {
                n137 = Index Array(array=w228, index=3) -> (element=w229:cluster{string[]})
                n138 = call <vilib>:"NT Read String.vi"("Name"=w231) -> ("String"=w230:string)  [unwired: 9 in, 1 out]
                n139 = Unbundle(w229) -> (w225:string[])
                n140 = Match First String(2:w225, 3:w230) -> (0:w226:i32)  [unwired: 1 out]
                n141 = property on="Test Ring" class="Ring (strict)"("Value"=w226, "Strings []"=w225) -> ()  [unwired: 2 in, 2 out]
                n142 = property on="Test Ring" class="Ring (strict)"("Visible"=TRUE) -> ()  [unwired: 2 in, 2 out]
                n143 = property on="Test Slider" class="Slide (strict)"("Visible"=FALSE) -> ()  [unwired: 2 in, 2 out]
              }
              frame "Color Enable  **" {
                n144 = Index Array(array=w237, index=4) -> (element=w238:cluster{string[]})
                n145 = call <vilib>:"NT Read String.vi"("Name"=w240) -> ("String"=w239:string)  [unwired: 9 in, 1 out]
                n146 = Unbundle(w238) -> (w234:string[])
                n147 = Match First String(2:w234, 3:w239) -> (0:w235:i32)  [unwired: 1 out]
                n148 = property on="Test Ring" class="Ring (strict)"("Value"=w235, "Strings []"=w234) -> ()  [unwired: 2 in, 2 out]
                n149 = property on="Test Ring" class="Ring (strict)"("Visible"=TRUE) -> ()  [unwired: 2 in, 2 out]
                n150 = property on="Test Slider" class="Slide (strict)"("Visible"=FALSE) -> ()  [unwired: 2 in, 2 out]
              }
              frame Default {
                n151 = property on="Test Ring" class="Ring (strict)"("Visible"=FALSE) -> ()  [unwired: 2 in, 2 out]
                n152 = property on="Test Slider" class="Slide (strict)"("Visible"=FALSE) -> ()  [unwired: 2 in, 2 out]
              }
              frame "Brightness  **", "Color Level  **", "Compression  **", "FPS  **", "Sharpness  **" {
                n153 = call <vilib>:"NT Read Number.vi"("Name"=w246) -> ("Numeric"=w245:dbl)  [unwired: 9 in, 1 out]
                n154 = local write "Test Slider"(w245) -> ()
                n155 = property on="Test Slider" class="Slide (strict)"("Visible"=TRUE, "Scale.Maximum"=100.0 ("Scale.Range:Maximum")) -> ()  [unwired: 2 in, 2 out]
                n156 = property on="Test Ring" class="Ring (strict)"("Visible"=FALSE) -> ()  [unwired: 2 in, 2 out]
              }
            }
          }
        }
        n157 = property on="Progress" class="Clust (strict)"("Visible"=FALSE) -> ()  [unwired: 2 in, 2 out]
      }
      event "Test Name": Mouse Enter {
        # "Populate the ring with the list of tests"
        n158 = event-data() -> ()  [unwired: 1 in, 1 out]
        n159 = call <vilib>:"NT Read String Array.vi"("Name"="TestMode/TestList") -> ("String Array"=w254:string[])  [unwired: 9 in, 1 out]
        n160 = Build Array (concatenate)("Select the test to run...", w254) -> (w253:string[])
        n161 = property on="Test Name" class="Ring (strict)"("Strings []"=w253) -> ()  [unwired: 2 in, 2 out]
      }
      event "Test Name": Value Change {
        w256 = FALSE ("Visible")
        # "Tell the robot the test name to run"
        n162 = event-data() -> ("NewVal"=w260:u16)  [unwired: 1 in]
        n163 = property on="Test Name" class="Ring (strict)"() -> ("Strings []"=w261:string[])  [unwired: 2 in, 2 out]
        n164 = local write "Progress"(T8 {"Test Progress"=0, "Test Progress Text"=""} ("Progress")) -> ()
        n165 = Index Array(array=w261, index=w260) -> (element=w259:string)
        n166 = call <vilib>:"NT Write String.vi"("String"=w259, "Name"="TestMode/TestName") -> ()  [unwired: 9 in, 1 out]
        n167 = property on="Progress" class="Clust (strict)"("Visible"=TRUE) -> ()  [unwired: 2 in, 2 out]
        n168 = property on="Motor" class="Clust (strict)"("Visible"=w256) -> ()  [unwired: 2 in, 2 out]
        n169 = property on="Test Slider" class="Slide (strict)"("Visible"=w256) -> ()  [unwired: 2 in, 2 out]
        n170 = property on="On/Off" class="Bool (strict)"("Visible"=w256) -> ()  [unwired: 2 in, 2 out]
        n171 = property on="Rev/Fwd" class="Clust (strict)"("Visible"=w256) -> ()  [unwired: 2 in, 2 out]
        n172 = property on="Test Ring" class="Ring (strict)"("Visible"=w256) -> ()  [unwired: 2 in, 2 out]
      }
      event "Listbox": Double Click {
        # "Shift clears all"
        # "Update symbols on the listbox"
        n173 = event-data() -> ("PlatMods.Shift"=w264:bool, "Row"=w266:i32)  [unwired: 1 in]
        n174 = case shown="True" w264 {
          tunnel: w266 -> [w270 _]
          tunnel: 1 -> [w269 _]
          frame False {
            n175 = property on="Listbox" class="LstBox (strict)"() -> ("Item Symbols"=w268:i32[])  [unwired: 2 in, 2 out]
            n176 = Replace Array Subset(array=w268, new element=w269, index=w270) -> (w267:i32[])
            n177 = property on="Listbox" class="LstBox (strict)"("Item Symbols"=w267) -> ()  [unwired: 2 in, 2 out]
          }
          frame True {
            w271 = 0 ("Top Row")
            n178 = property on="Listbox" class="LstBox (strict)"() -> ("Number of Rows"=w273:u32)  [unwired: 2 in, 2 out]
            n179 = Initialize Array(0, w273) -> (w272:i32[])
            n180 = property on="Listbox" class="LstBox (strict)"("Top Row"=w271, "Value"=w271, "Item Symbols"=w272) -> ()  [unwired: 2 in, 2 out]
          }
        }
      }
      event "Listbox": Key Down {
        # "Update symbols on the listbox\nLeft and right keys check and uncheck"
        n181 = event-data() -> ("VKey"=w277:T20)  [unwired: 1 in]
        n182 = case shown="\"Left\", \"Right\"" w277 {
          selector: w277 -> [w282 _]
          tunnel: eventvkey."Left" ("VKey") -> [w280 _]
          frame "Left", "Right" {
            n183 = Equal?(x=w280, y=w282) -> (x = y?=w281:bool)
            n184 = Select(t=0, s=w281, f=1) -> (s? t:f=w283:i32)
            n185 = property on="Listbox" class="LstBox (strict)"() -> ("Item Symbols"=w286:i32[])  [unwired: 2 in, 2 out]
            n186 = Replace Array Subset(array=w286, new element=w283, index="Listbox") -> (w285:i32[])
            n187 = property on="Listbox" class="LstBox (strict)"("Item Symbols"=w285) -> ()  [unwired: 2 in, 2 out]
          }
          frame Default {
          }
        }
      }
      event "DB Camera Config": Value Change {
        # "Show or hide the cluster of controls, store in ini file"
        n188 = event-data() -> ("NewVal"=w290:bool)  [unwired: 1 in]
        n189 = case shown="False" w290 {
          tunnel: w289 -> [w299 _]
          tunnel: [w292 w310] -> w288
          tunnel: w287 -> [w291 w310]
          frame False {
            w306 = "Camera"
            w309 = FALSE ("Visible")
            n190 = local read "Camera Settings"() -> (w298:T3)
            n191 = Index Array(array=w299) -> (element=w302:cluster{string[]})  [unwired: 1 in]
            n192 = Unbundle(w298) -> ("Frame Rate"=w297:i32, "Compression"=w296:i32, "Size"=w300:u16)
            n193 = Unbundle(w302) -> (w301:string[])
            n194 = Index Array(array=w301, index=w300) -> (element=w295:string)
            n195 = call-poly <vilib>:"Write Key.vi"("section"=w306, "value"=w295, "key"="Size", "refnum"=w291) -> ("refnum out"=w308:T18)  [unwired: 2 in, 5 out]
            n196 = call-poly <vilib>:"Write Key.vi"("section"=w306, "value"=w297, "key"="FrameRate", "refnum"=w308) -> ("refnum out"=w307:T18)  [unwired: 1 in, 6 out]
            n197 = property on="Camera Settings" class="Clust (strict)"("Visible"=w309) -> ()  [unwired: 2 in, 2 out]
            n198 = local write "DB Camera Config"(w309) -> ()
            n199 = call-poly <vilib>:"Write Key.vi"("section"=w306, "value"=w296, "key"="Compression", "refnum"=w307) -> ("refnum out"=w293:T18)  [unwired: 1 in, 6 out]
            n200 = call <vilib>:"Close Config Data.vi"("refnum"=w293) -> ("file path"=w294:path)  [unwired: 2 in, 8 out]
            n201 = call <vilib>:"Open Config Data.vi"("configuration file path"=w294) -> ("refnum"=w292:T18)  [unwired: 8 in, 2 out]
          }
          frame True {
            n202 = property on="Camera Settings" class="Clust (strict)"("Visible"=TRUE) -> ()  [unwired: 2 in, 2 out]
          }
        }
      }
      event "Camera Settings": Value Change {
        # "Update summary string when any elements of DB camera change"
        n203 = event-data() -> ("NewVal"=w323:T3)  [unwired: 1 in]
        n204 = Index Array(array=w319) -> (element=w318:cluster{string[]})  [unwired: 1 in]
        n205 = Unbundle(w323) -> ("Frame Rate"=w314:i32, "Compression"=w313:i32, "Size"=w316:u16)
        n206 = Unbundle(w318) -> (w317:string[])
        n207 = Index Array(array=w317, index=w316) -> (element=w315:string)
        n208 = Format Into String(format string="%s   %dfps   %d%%", w315, w314, w313) -> (resulting string=w320:string)  [unwired: 2 in, 1 out]
        n209 = Build Array(w320) -> (w321:string[])
        n210 = property on="DB Camera Config" class="Bool (strict)"("Strings [4]"=w321) -> ()  [unwired: 2 in, 2 out]
      }
      event "Motor.Enable": Value Change {
        # "When the test mode otor enable helper is set, update that\ntree row item's value"
        n211 = event-data() -> ("NewVal"=w329:bool)  [unwired: 1 in]
        n212 = Unbundle("Motor") -> ("Value"=w328:dbl)  [unwired: 1 out]
        n213 = Select(t=w328, s=w329, f=0.0) -> (s? t:f=w326:dbl)
        n214 = call <vilib>:"NT Write Number.vi"("Numeric"=w326, "Name"=w325) -> ()  [unwired: 9 in, 1 out]
      }
      event "Test Slider": Value Change {
        # "When the test mode slider helper is set, update that\ntree row item's value"
        n215 = event-data() -> ("NewVal"=w332:dbl)  [unwired: 1 in]
        n216 = call <vilib>:"NT Write Number.vi"("Numeric"=w332, "Name"=w333) -> ()  [unwired: 9 in, 1 out]
      }
      event "On/Off": Value Change {
        # "When the test mode on/off helper value is set, update that\ntree row item's value"
        n217 = event-data() -> ("NewVal"=w337:bool)  [unwired: 1 in]
        n218 = Boolean To (0,1)(Boolean=w337) -> (0, 1=w336:i16)
        n219 = call <vilib>:"NT Write Number.vi"("Numeric"=w336, "Name"=w335) -> ()  [unwired: 9 in, 1 out]
      }
      event "Rev/Fwd": Value Change {
        # "When the test mode helper value for relays is set, update that\ntree row item's value"
        n220 = event-data() -> ("NewVal.Forward"=w345:bool, "NewVal.Reverse"=w344:bool)  [unwired: 1 in]
        n221 = Boolean To (0,1)(Boolean=w345) -> (0, 1=w341:i16)
        n222 = Boolean To (0,1)(Boolean=w344) -> (0, 1=w343:i16)
        n223 = Negate(x=w343) -> (-x=w342:i16)
        n224 = Add(x=w341, y=w342) -> (x+y=w340:i16)
        n225 = call <vilib>:"NT Write Number.vi"("Numeric"=w340, "Name"=w339) -> ()  [unwired: 9 in, 1 out]
      }
      event "Test Ring": Value Change {
        # "When a test mode helper value is selected from the ring,\nset the tree item's variable to the string value"
        n226 = event-data() -> ("NewVal"=w349:u16)  [unwired: 1 in]
        n227 = property on="Test Ring" class="Ring (strict)"() -> ("Strings []"=w350:string[])  [unwired: 2 in, 2 out]
        n228 = Index Array(array=w350, index=w349) -> (element=w348:string)
        n229 = call <vilib>:"NT Write String.vi"("String"=w348, "Name"=w347) -> ()  [unwired: 9 in, 1 out]
      }
      event "Rec Mode": Value Change {
        # "Update globals for recording mode and path to read log from.\nClear when logging and let NetworkTables set path for vision to\nuse."
        n230 = event-data() -> ("NewVal"=w360:enum32{"Stop", "Record", "Playback"})  [unwired: 1 in]
        n231 = global write "WPI_DashboardLogging Global.vi" "Logging Filename"(path "") -> ()
        n232 = case shown="\"Playback\"" w360 {
          tunnel: w359 -> [_ w362 w370]
          tunnel: [_ _ w369] -> w356
          tunnel: [_ _ w368] -> _
          tunnel: w354 -> [_ _ w366]
          tunnel: cluster{i32, i32} {-250, 170} -> [_ _ w365]
          tunnel: [_ _ T21 {"Image Size"=TRUE, "Image Type"=TRUE, "Pixel Value"=TRUE, "ROI Information"=TRUE, "Zoom Factor"=FALSE} ("Image Information Shown:All Elements")] -> w352
          tunnel: [_ _ TRUE ("Zoom Factor")] -> w351
          frame Default {
          }
          frame "Stop", "Record" {
            # "Place Window too"
            n233 = invoke class="VI" method="FP.Close"(reference=w362) -> (reference out=w361:refnum<vi>)  [unwired: 2 in, 2 out]
            n234 = invoke class="VI" method="Abort VI"(reference=w361) -> ()  [unwired: 2 in, 3 out]
          }
          frame "Playback" {
            n235 = call "Open Playback Panel.vi"("Offset"=w365, "DB VI Ref"=w366, "Playback in"=w370) -> ("Playback out"=w367:refnum<vi>)  [unwired: 8 in]
            n236 = register-events(w367) -> (reference out=w369:refnum<event-registration>, error out=w368:errorcluster)  [unwired: 2 in]
          }
        }
        n237 = global write "WPI_DashboardLogging Global.vi" "Recording"(w360) -> ()
        n238 = property on="Big" class="ImageControl"("Image Information Shown"=w352, "Image Information Visible"=w351) -> ()  [unwired: 2 in, 2 out]
        n239 = call <vilib>:"WPI_DashboardNT Log FieldName Cache.vi"("Operation"=enum16{"Lookup/Add", "Index", "Clear"}."Clear") -> ()  [unwired: 8 in, 3 out]
      }
      event Panel Close {
        w371 = enum32{"Stop", "Record", "Playback"}."Stop" ("Rec Mode")
        # "Playback window has been closed, abort"
        n240 = event-data() -> ()  [unwired: 1 in, 4 out]
        n241 = local write "Rec Mode"(w371) -> ()
        n242 = global write "WPI_DashboardLogging Global.vi" "Recording"(w371) -> ()
      }
      event Panel Close {
        # "Abort playback window and ourself"
        n243 = event-data() -> ()  [unwired: 1 in, 4 out]
        n244 = invoke class="VI" method="FP.Close"(reference=w376) -> (reference out=w375:refnum<vi>)  [unwired: 2 in, 2 out]
        n245 = invoke class="VI" method="Abort VI"(reference=w375) -> (error out=w374:errorcluster)  [unwired: 2 in, 2 out]
        n246 = invoke class="VI" method="Abort VI"(error in=w374) -> ()  [unwired: 2 in, 3 out]
      }
      event "Vision": Value Change {
        # "Enable/Disable Compression slider.\nHW USB is hard-coded into the camera"
        n247 = event-data() -> ("NewVal"=w382:u16)  [unwired: 1 in]
        n248 = Equal?(x=w382, y=u32 2 ("milliseconds to wait")) -> (x = y?=w380:bool)
        n249 = Select(t=T22."Disabled and Grayed Out" ("Disabled"), s=w380, f=T22."Enabled" ("Disabled")) -> (s? t:f=w377:T22)
        n250 = property on="Compression" class="Slide (strict)"("DisabledEnum"=w377) -> ()  [unwired: 2 in, 2 out]
      }
    }
  }
  n251 = while {
    tunnel: w43 -> [w385]
    i -> [w388]
    stop <- FALSE stop-if-true
    n252 = Wait (ms)(milliseconds to wait=u32 100) -> ()  [unwired: 1 out]
    n253 = case shown="\"Playback\"" "Rec Mode" {
      tunnel: w388 -> [_ _ w403]
      tunnel: [u32 2829099 ("Base Color") u32 11141120 ("Target Color") w392] -> w384
      frame "Stop", Default {
        # "Reset the color, extra updates don't cost much"
      }
      frame "Record" {
      }
      frame "Playback" {
        # "Playback"
        n254 = Quotient & Remainder(x=w403, y=u32 50 ("milliseconds to wait")) -> (x-y*floor(x/y)=w399:u32)  [unwired: 1 out]
        n255 = Divide(x=w399, y=u32 50 ("milliseconds to wait")) -> (x/y=w396:dbl)
        n256 = Multiply(x=6.283185307179586, y=w396) -> (x*y=w401:dbl)
        n257 = Sine(x=w401) -> (sin(x)=w400:dbl)
        n258 = Absolute Value(x=w400) -> (abs(x)=w393:dbl)
        n259 = call "Interpolate RGB Color.vi"("Proportion"=w393, "Target Color"=u32 30976, "Base Color"=u32 2829099) -> ("Result Color"=w392:u32)  [unwired: 8 in]
      }
    }
    n260 = property class="Pane"(reference=w385, "PaneColor"=w384) -> ()  [unwired: 1 in, 2 out]
  }
  n261 = TCP Create Listener(10:u16 1741 ("timeout ms (25000)")) -> (3:w6:refnum<k5>)  [unwired: 4 in, 2 out]
  n262 = while {
    tunnel: w6 -> [w405]
    stop <- FALSE stop-if-true
    n263 = TCP Wait On Listener(11:w405) -> (4:w404:refnum<k5>)  [unwired: 3 in, 4 out]
    n264 = local write "TCP"(w404) -> ()
  }
  n265 = property on="On/Off" class="Bool (strict)"("Visible"=w11) -> ()  [unwired: 2 in, 2 out]
  n266 = property on="Motor" class="Clust (strict)"("Visible"=w11) -> ()  [unwired: 2 in, 2 out]
  n267 = property on="Progress" class="Clust (strict)"("Visible"=w11) -> ()  [unwired: 2 in, 2 out]
  n268 = property on="Test Ring" class="Ring (strict)"("Visible"=w11) -> ()  [unwired: 2 in, 2 out]
  n269 = property on="Rev/Fwd" class="Clust (strict)"("Visible"=w11) -> ()  [unwired: 2 in, 2 out]
  n270 = property on="Camera Settings" class="Clust (strict)"("Visible"=w11) -> ()  [unwired: 2 in, 2 out]
  n271 = local write "DB Camera Config"(w11) -> ()
  n272 = global write "WPI_DashboardLogging Global.vi" "Recording"(w37) -> ()
  n273 = local write "Rec Mode"(w37) -> ()
  n274 = local write "Axis Cam IP"("10.44.18.11" ("Axis Cam IP")) -> ()
  n275 = call "IMAQ Create"("Image Name"="Dashboard Image", "Image Type"=w57) -> ("New Image"=w55:T1, "error out"=w54:errorcluster)  [unwired: 2 in, 1 out]
  n276 = call "IMAQ Create"("Image Name"="Dashboard Image", "Image Type"=w4) -> ("New Image"=w3:T1, "error out"=w2:errorcluster)  [unwired: 2 in, 1 out]
  n277 = while {
    tunnel: w55 -> [w426]
    tunnel: w54 -> [_]
    tunnel: [w427] -> _
    tunnel: w3 -> [w410]
    tunnel: w2 -> [_]
    i -> [w427]
    stop <- FALSE stop-if-true
    (unwired) FALSE
    # "Optionally read the DB image,\nlog, or retrieve images from a\nlogged match"
    # "Optionally read the DB image,\nlog, or retrieve images from a\nlogged match"
    n278 = case shown="False" "Enable" {
      tunnel: [w431 w432] -> w418
      frame False {
        w431 = u16 0 items=["Camera Off", "USB Camera SW", "USB Camera HW", "IP Camera"] ("Vision")
      }
      frame True {
        w432 = u16 1 items=["Camera Off", "USB Camera SW", "USB Camera HW", "IP Camera"] ("Vision")
      }
    }
    n279 = local read "Rec Mode"() -> (w409:enum32{"Stop", "Record", "Playback"})
    n280 = local read "Rec Mode"() -> (w420:enum32{"Stop", "Record", "Playback"})
    n281 = local read "Camera IP"() -> (w419:string)
    n282 = local read "Camera Settings"() -> (w417:T3)
    n283 = case shown="False" "Enable" {
      tunnel: [w429 w430] -> w416
      frame False {
        w429 = u16 0 items=["Camera Off", "USB Camera SW", "USB Camera HW", "IP Camera"] ("Vision")
      }
      frame True {
        w430 = u16 3 items=["Camera Off", "USB Camera SW", "USB Camera HW", "IP Camera"] ("Vision")
      }
    }
    n284 = call <vilib>:"WPI_CameraRead MJPG for Dashboard.vi"("Camera Settings"="Camera Settings", "Rec Mode"=w420, "Camera IP"=w419, "Camera Mode"=w418, "Refnum in"=w426) -> ("Active"=w424:bool, "Refnum out"=w425:T1, "FPS"=w423:dbl, "Bandwidth (Mbps)"=w422:dbl)  [unwired: 3 in]
    n285 = call <vilib>:"WPI_CameraRead MJPG for Dashboard.vi"("Camera Settings"=w417, "Rec Mode"=w409, "Camera IP"="Axis Cam IP", "Camera Mode"=w416, "Refnum in"=w410) -> ("Active"=w412:bool, "Refnum out"=w411:T1, "FPS"=w413:dbl, "Bandwidth (Mbps)"=w414:dbl)  [unwired: 3 in]
    n286 = case shown="True" w424 {
      tunnel: w425 -> [_ w454]
      tunnel: w422 -> [_ w453]
      tunnel: w423 -> [_ w452]
      tunnel: "Toggle" -> [_ w450]
      frame False {
        # "Sleep for 500ms"
        n287 = Wait Until Next ms Multiple(millisecond multiple=u32 500) -> ()  [unwired: 1 out]
      }
      frame True {
        # "Here is where you would annotate,\npossibly process, and display the image"
        # "Update Mbps LED"
        n288 = call "IMAQ Clear Overlay"("Image"=w454) -> ("error out"=w458:errorcluster, "Image Out"=w451:T1)  [unwired: 2 in, 7 out]
        n289 = case shown="4, 5" w453 {
          tunnel: [u32 6618880 ("Color Box") u32 16776722 ("Color Box") u32 16716800 ("Color Box")] -> w455
          frame Default {
          }
          frame 4, 5 {
          }
          frame 6.. {
          }
        }
        n290 = Unbundle By Name(w458) -> ("status"=w459:bool)
        n291 = Bundle("Color Box"=w455, "Color Box"=w455) -> (w457:cluster{"Color Box":u32, "Color Box":u32})  [unwired: 1 out]
        n292 = property on="Image Message" class="Str"("Visible"=w459) -> ()  [unwired: 2 in, 2 out]
        n293 = Build Array(w457) -> (w456:cluster{"Color Box":u32, "Color Box":u32}[])
        n294 = property on="Mbps 2" class="Bool (strict)"("Colors [4]"=w456) -> ()  [unwired: 2 in, 2 out]
        n295 = case shown="False" w450 {
          tunnel: w451 -> [w460 w461]
          frame False {
            n296 = local write "Big"(w460) -> ()
          }
          frame True {
            n297 = local write "Small"(w461) -> ()
          }
        }
        "Mbps" <- w453
        "fps" <- w452
      }
    }
    n298 = case shown="True" w412 {
      tunnel: w411 -> [_ w438]
      tunnel: w414 -> [_ w436]
      tunnel: w413 -> [_ w437]
      tunnel: "Toggle" -> [_ w434]
      frame False {
        # "Sleep for 500ms"
        n299 = Wait Until Next ms Multiple(millisecond multiple=u32 500) -> ()  [unwired: 1 out]
      }
      frame True {
        # "Here is where you would annotate,\npossibly process, and display the image"
        # "Update Mbps LED"
        n300 = call "IMAQ Clear Overlay"("Image"=w438) -> ("error out"=w442:errorcluster, "Image Out"=w435:T1)  [unwired: 2 in, 7 out]
        n301 = case shown="4, 5" w436 {
          tunnel: [u32 6618880 ("Color Box") u32 16776722 ("Color Box") u32 16716800 ("Color Box")] -> w439
          frame Default {
          }
          frame 4, 5 {
          }
          frame 6.. {
          }
        }
        n302 = Unbundle By Name(w442) -> ("status"=w443:bool)
        n303 = Bundle("Color Box"=w439, "Color Box"=w439) -> (w441:cluster{"Color Box":u32, "Color Box":u32})  [unwired: 1 out]
        n304 = property on="Image Message" class="Str"("Visible"=w443) -> ()  [unwired: 2 in, 2 out]
        n305 = Build Array(w441) -> (w440:cluster{"Color Box":u32, "Color Box":u32}[])
        n306 = property on="Mbps 3" class="Bool (strict)"("Colors [4]"=w440) -> ()  [unwired: 2 in, 2 out]
        n307 = case shown="False" w434 {
          tunnel: w435 -> [w444 w445]
          frame False {
            n308 = local write "Small"(w444) -> ()
          }
          frame True {
            n309 = local write "Big"(w445) -> ()
          }
        }
        "fps 2" <- w437
        "Mbps 4" <- w436
      }
    }
  }
